vi "encode-to-json.vi"(8 "Sensor Options":T1={"Display Units"="units", "Zero Offset"=2.62, "Sensor Min"=0.0, "Sensor Max"=500.0, "Signal Min"=0.0, "Signal Max"=100.0, "Conversion Factor"=0.0}, 9 "Serial Port Options":T2={"COM Port (COM10)"="COM10", "baud rate (19200)"=19200, "Simulate Hardware"=FALSE} {"baud rate (19200)" max=115200 step=1200}, 10 "Datalogging options":T3={"data-precision"=3, "Include Date"=FALSE, "Include Timestamp"=TRUE, "Include Milliseconds"=FALSE, "sample-rate (Hz)"=4.0, "Logging Active"=TRUE}, 11 "Filepath Selection":T4={"Log Filepath Source"=enum."Application Relative (Auto)", "Log File Path (Manual)"=path "C:/Users/dheard/Documents/0002-labview-projects/ammonia-absorbsion-rig/data", "Log File Folder Name"="data", "log file name"="log", "Include Date in Filename"=TRUE, "Include Time in Filename"=TRUE}) -> (0 "sensor-options-json":string, 1 "serial-port-json":string, 2 "data-logging-json":string, 3 "filepath-json":string)   [LabVIEW 2024]
uses:
  utils-sub-vi/csv-file-logging-util/filepath-selection.ctl
  utils-sub-vi/csv-file-logging-util/datalogging-options.ctl
  serial-options.ctl
  sensor-options.ctl
  filepath-json-cluster-feck.ctl
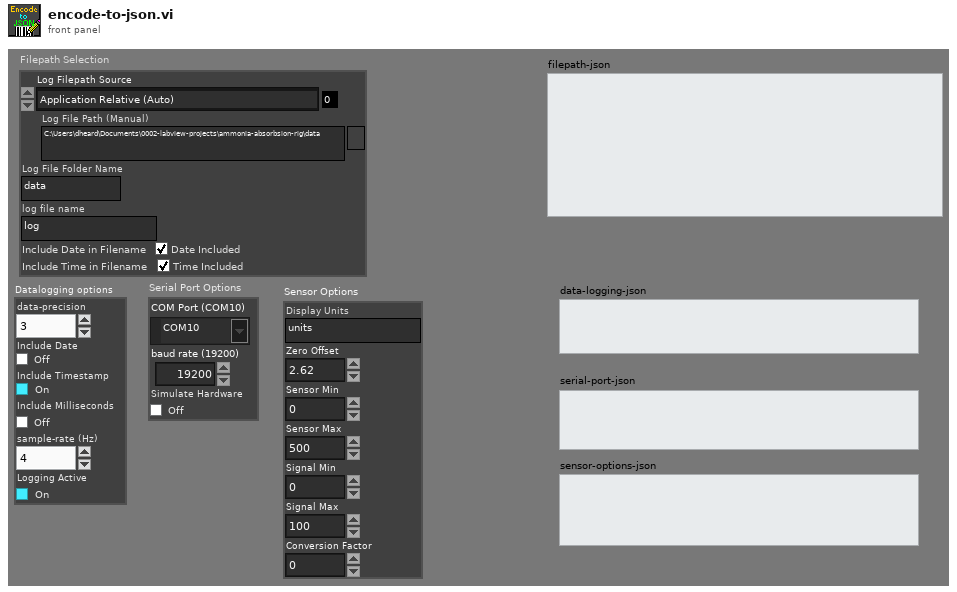
[diagram p1: front panel]
types:
  T1 = typedef "sensor-options.ctl" = cluster{"Display Units":string, "Zero Offset":dbl, "Sensor Min":dbl, "Sensor Max":dbl, "Signal Min":dbl, "Signal Max":dbl, "Conversion Factor":dbl}
  T2 = typedef "serial-options.ctl" = cluster{"COM Port (COM10)":refnum<visa-resource-name>, "baud rate (19200)":u32, "Simulate Hardware":bool}
  T3 = typedef "datalogging-options.ctl" = cluster{"data-precision":i32, "Include Date":bool, "Include Timestamp":bool, "Include Milliseconds":bool, "sample-rate (Hz)":dbl, "Logging Active":bool}
  T4 = typedef "filepath-selection.ctl" = cluster{"Log Filepath Source":enum16{"Application Relative (Auto)", "VI Relative (Auto)", "Complete Path (Manual)"}, "Log File Path (Manual)":path, "Log File Folder Name":string, "log file name":string, "Include Date in Filename":bool, "Include Time in Filename":bool}
  T5 = typedef "filepath-json-cluster-feck.ctl" = cluster{"Log Filepath Source":i32, "Log Filepath byte array":u8[], "Log File Folder Name":string, "log file name":string, "Include Date in Filename":bool, "Include Time in Filename":bool}
  T6 = enum16{"Application Relative (Auto)", "VI Relative (Auto)", "Complete Path (Manual)"}
  T7 = cluster{"unsigned byte array":u8[], "baud rate (19200)":u32, "Simulate Hardware":bool}
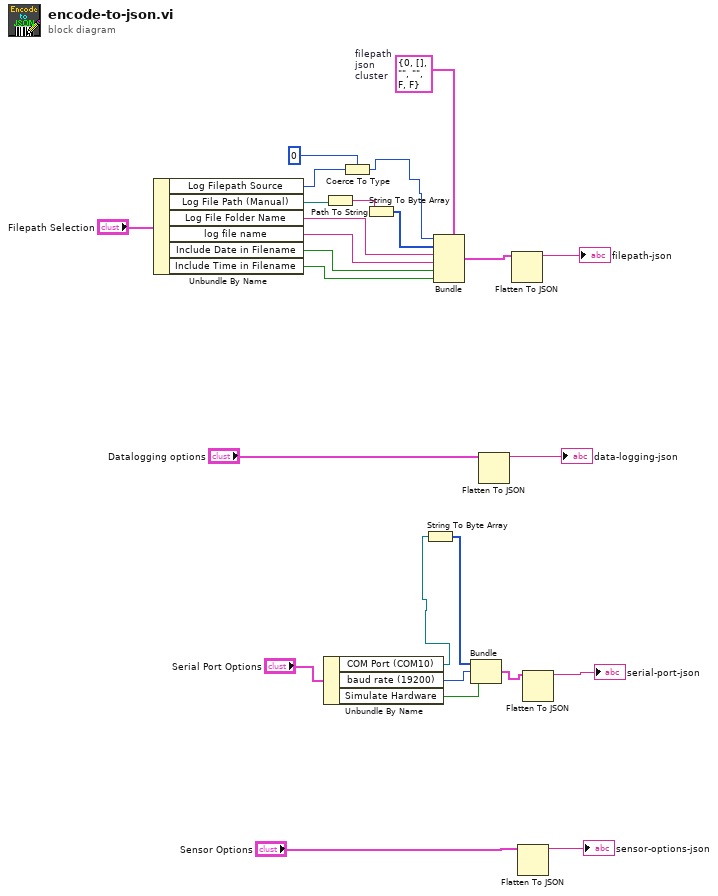
[diagram p0: block diagram]
diagram:
  w7 = T5 {"Log Filepath Source"=0, "Log Filepath byte array"=[], "Log File Folder Name"="", "log file name"="", "Include Date in Filename"=FALSE, "Include Time in Filename"=FALSE}  # filepath json cluster
  n1 = Unbundle By Name("Filepath Selection") -> ("Log Filepath Source"=w9:T6, "Log File Path (Manual)"=w8:path, "Log File Folder Name"=w25:string, "log file name"=w24:string, "Include Date in Filename"=w23:bool, "Include Time in Filename"=w22:bool)
  n2 = Unbundle By Name("Serial Port Options") -> ("COM Port (COM10)"=w3:refnum<visa-resource-name>, "baud rate (19200)"=w19:u32, "Simulate Hardware"=w18:bool)
  n3 = Path To String(path=w8) -> (string=w13:string)
  n4 = Coerce To Type(0:w9, 1:0) -> (2:w5:i32)
  n5 = String To Byte Array(string=w13) -> (unsigned byte array=w12:u8[])
  n6 = String To Byte Array(string=w3) -> (unsigned byte array=w2:u8[])
  n7 = Bundle(cluster=w7, "Log Filepath Source"=w5, "Log Filepath byte array"=w12, "Log File Folder Name"=w25, "log file name"=w24, "Include Date in Filename"=w23, "Include Time in Filename"=w22) -> (w6:T5)
  n8 = Bundle("unsigned byte array"=w2, "baud rate (19200)"=w19, "Simulate Hardware"=w18) -> (w20:T7)  [unwired: 1 in]
  n9 = Flatten To JSON(anything="Datalogging options") -> (JSON string=→"data-logging-json":string)  [unwired: 2 in, 1 out]
  n10 = Flatten To JSON(anything=w6) -> (JSON string=→"filepath-json":string)  [unwired: 2 in, 1 out]
  n11 = Flatten To JSON(anything="Sensor Options") -> (JSON string=→"sensor-options-json":string)  [unwired: 2 in, 1 out]
  n12 = Flatten To JSON(anything=w20) -> (JSON string=→"serial-port-json":string)  [unwired: 2 in, 1 out]
